vi "Charger_Next_Action.vi"(5 "Setpoint":dbl=nan, 6 "error in":errorcluster, 7 "ReceivedLevel":dbl=nan format="%.1f", 8 "Temperature":dbl=nan, 9 "ChargingState":string="CHARGE_CC_FAST-2") -> (0 "error out":errorcluster, 1 "Adjustment":dbl=nan, 2 "Charger":T1=enum."na", 4 "Match":bool)   [LabVIEW 2020]
uses:
  Charger_Next_Action.ctl
  Charger_States_Control.ctl
panel:
  out "index":i32=-1
  in  "Charge Decision":T2[](array[typedef])=[{"ChargingState"="Any", "Temp"=enum."GT 3", "Low Limit"=inf, "High Limit"=-inf, "Charger"=enum."Pause", "Adjustment"=0.0}, {"ChargingState"="CHARGE_OFF-0", "Temp"=enum."LE 3", "Low Limit"=inf, "High Limit"=225.0, "Charger"=enum."Adjust", "Adjustment"=-100.0}, {"ChargingState"="CHARGE_OFF-0", "Temp"=enum."LE 3", "Low Limit"=200.0, "High Limit"=25.0, "Charger"=enum."Adjust", "Adjustment"=100.0}, {"ChargingState"="CHARGE_OFF-0", "Temp"=enum."LE 3", "Low Limit"=25.0, "High Limit"=-inf, "Charger"=enum."Enable", "Adjustment"=0.0}, {"ChargingState"="CHARGE_PRE_CONDITION-1", "Temp"=enum."LE 3", "Low Limit"=inf, "High Limit"=225.0, "Charger"=enum."Adjust", "Adjustment"=-100.0}, {"ChargingState"="CHARGE_PRE_CONDITION-1", "Temp"=enum."LE 3", "Low Limit"=200.0, "High Limit"=-inf, "Charger"=enum."Adjust", "Adjustment"=100.0}, {"ChargingState"="CHARGE_CC_FAST-2", "Temp"=enum."LE 3", "Low Limit"=inf, "High Limit"=150.0, "Charger"=enum."Adjust", "Adjustment"=-100.0}, {"ChargingState"="CHARGE_CC_FAST-2", "Temp"=enum."LE 3", "Low Limit"=130.0, "High Limit"=-inf, "Charger"=enum."Adjust", "Adjustment"=100.0}, {"ChargingState"="CHARGE_CC_SLOW-3", "Temp"=enum."GT 2", "Low Limit"=inf, "High Limit"=150.0, "Charger"=enum."Adjust", "Adjustment"=-100.0}, {"ChargingState"="CHARGE_CC_SLOW-3", "Temp"=enum."GT 2", "Low Limit"=130.0, "High Limit"=-inf, "Charger"=enum."Adjust", "Adjustment"=100.0}, {"ChargingState"="CHARGE_CC_SLOW-3", "Temp"=enum."LE 2", "Low Limit"=inf, "High Limit"=225.0, "Charger"=enum."Adjust", "Adjustment"=-100.0}, {"ChargingState"="CHARGE_CC_SLOW-3", "Temp"=enum."LE 2", "Low Limit"=200.0, "High Limit"=-inf, "Charger"=enum."Adjust", "Adjustment"=100.0}, {"ChargingState"="CHARGE_COMPLETE-4", "Temp"=enum."Any", "Low Limit"=inf, "High Limit"=-inf, "Charger"=enum."Disable", "Adjustment"=0.0}, {"ChargingState"="CHARGE_ERROR-5", "Temp"=enum."Any", "Low Limit"=inf, "High Limit"=-inf, "Charger"=enum."Disable", "Adjustment"=0.0}] {"High Limit" format="%.1f"; "Low Limit" format="%.1f"; "Adjustment" format="%.1f"}
  # "Low Limit"
  # "High Limit"
  # "ChargingState"
  # "Temp"
  # "Charger"
  # "Adjustment"
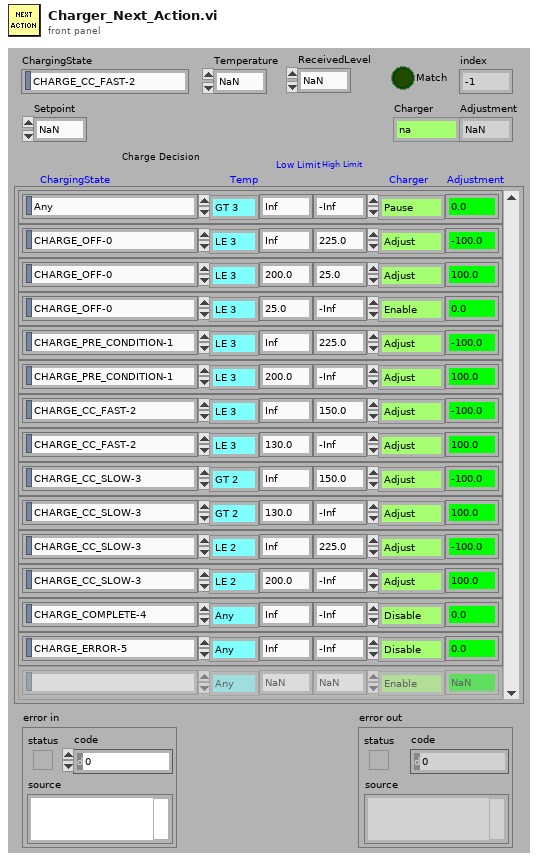
[diagram p1: front panel]
types:
  T1 = typedef "Charger_States_Control.ctl" = enum16{"Enable", "Disable", "Adjust", "Pause", "na"}
  T2 = typedef "Charger_Next_Action.ctl" = cluster{"ChargingState":string, "Temp":enum16{"Any", "GT 3", "LE 3", "GT 2", "LE 2"}, "Low Limit":dbl, "High Limit":dbl, "Charger":T1, "Adjustment":dbl}
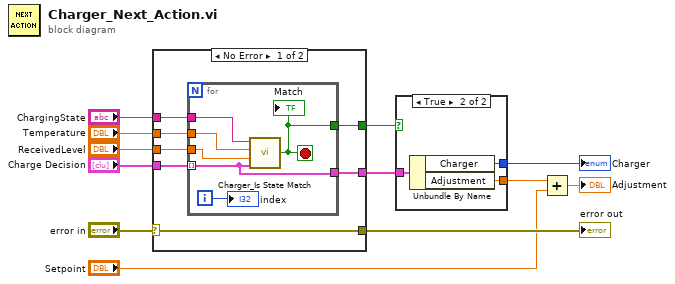
[diagram p0: block diagram]
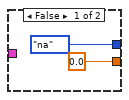
[diagram p2: hidden frame]
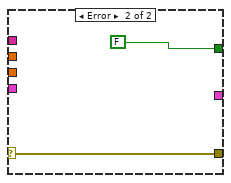
[diagram p3: hidden frame]
diagram:
  n1 = case shown="No Error" "error in" {
    selector: "error in" -> [w15 w27]
    tunnel: "Charge Decision" -> [w19 _]
    tunnel: "ReceivedLevel" -> [w18 _]
    tunnel: "Temperature" -> [w17 _]
    tunnel: "ChargingState" -> [w16 _]
    tunnel: [w15 w27] -> w7
    tunnel: [w14 _] -> w6
    tunnel: [w13 FALSE ("Match")] -> w5
    frame No Error {
      n2 = for {
        tunnel: w19 -> [w22] mode=indexing
        tunnel: w18 -> [w25]
        tunnel: w17 -> [w24]
        tunnel: w16 -> [w23]
        tunnel: [w22] -> w14
        tunnel: [w21] -> w13
        i -> [w20]
        stop <- w21 stop-if-true
        n3 = call "Charger_Is State Match.vi"("ChargeRecord"=w22, "ReceivedLevel"=w25, "TemperatureLevel"=w24, "ChargingState"=w23) -> ("Match"=w21:bool)
        "Match" <- w21
        "index" <- w20
      }
    }
    frame Error {
    }
  }
  "error out" <- w7
  n4 = case shown="True" w5 {
    tunnel: w6 -> [_ w32]
    tunnel: [Charger_States_Control."na" ("Charger") w31] -> w4
    tunnel: [0.0 ("Adjustment") w30] -> w2
    frame False {
    }
    frame True {
      n5 = Unbundle By Name(w32) -> ("Charger"=w31:T1, "Adjustment"=w30:dbl)
    }
  }
  "Charger" <- w4
  n6 = Add(x=w2, y="Setpoint") -> (x+y=→"Adjustment":dbl)
